vi "Write Requirements Path.vi"(10 "URI":string, 11 "Project in":refnum<class "TraceabilityMatrix.lvclass">) -> (3 "Project out":refnum<class "TraceabilityMatrix.lvclass">)   [LabVIEW 2021, in "Bananas.lvlib" / "TraceabilityMatrix.lvclass"]
uses:
  TraceabilityMatrix.lvclass
  TraceabilityMatrix.lvclass/TraceabilityMatrix.ctl
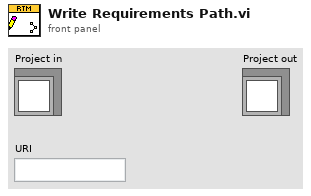
[diagram p1: front panel]
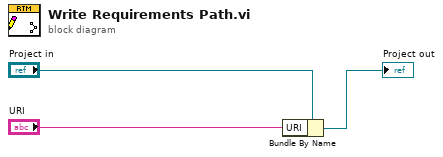
[diagram p0: block diagram]
diagram:
  n1 = Bundle By Name(cluster="Project in", "URI"="URI") -> (→"Project out":refnum<class "TraceabilityMatrix.lvclass">)
